vi "Get Nesting Test Project Path.vi"(11 "LUnit Test Suite Tests in":refnum<class "Test FInder Test.lvclass">) -> (3 "appended path":path)   [LabVIEW 2020, in "Test FInder Test.lvclass"]
uses:
  Test FInder Test.lvclass
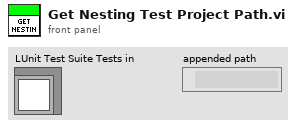
[diagram p1: front panel]
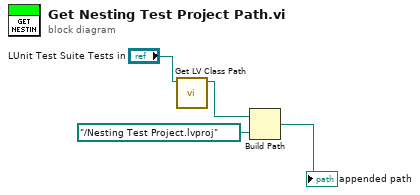
[diagram p0: block diagram]
diagram:
  n1 = call <vilib>:"Get LV Class Path.vi"("object"="LUnit Test Suite Tests in") -> ("class path"=w2:path)  [unwired: 9 in, 1 out]
  n2 = Build Path(base path=w2, name or relative path=path "../Nesting Test Project.lvproj") -> (appended path=→"appended path":path)
